vi "SC_schleife_init_JT_2.vi"   [LabVIEW 2016]
uses:
  Global/Global Variables/global.vi
  Global/Global Variables/Data_Display_global.vi
  Instrument_Setup.vi
types:
  T1 = typedef "PSIO.ctl" = cluster{"Address":T2, "Version":enum16{"PS", "IPS"}}
  T2 = typedef "OxfordAddress.ctl" = cluster{"Com Port":i32, "ISOBUS Address":i32, "GPIB Address":i16, "Communication":enum16{"RS232", "ISOBUS", "GPIB", "Gateway"}}
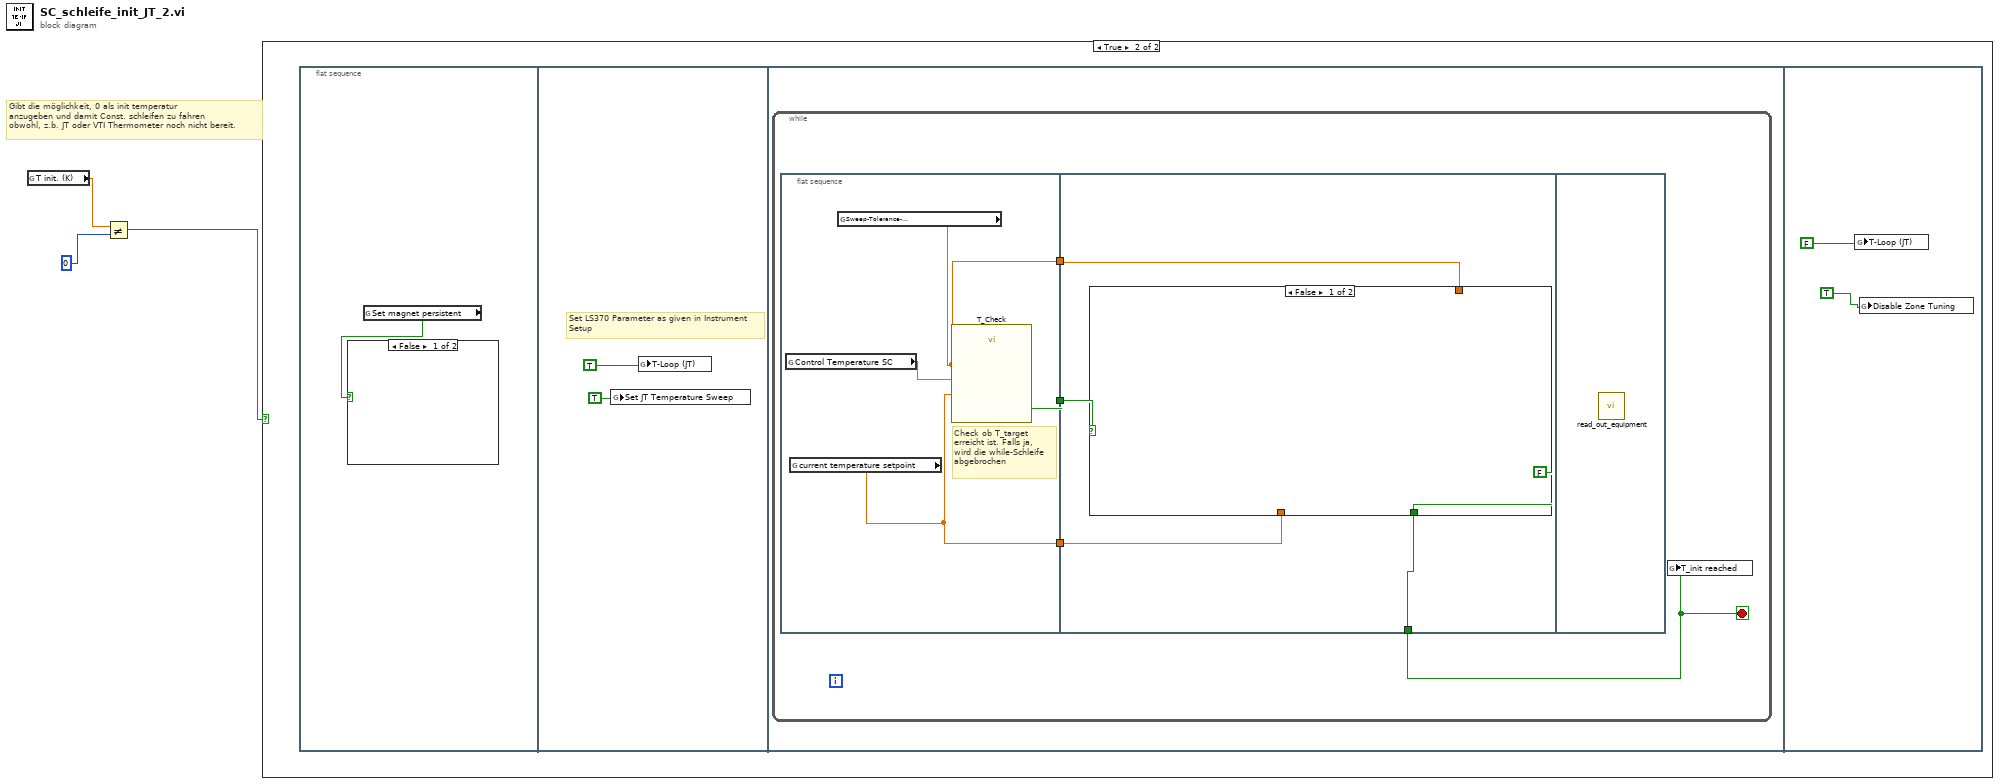
[diagram p0: block diagram]
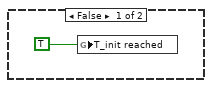
[diagram p2: hidden frame]
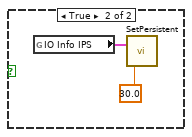
[diagram p3: hidden frame]
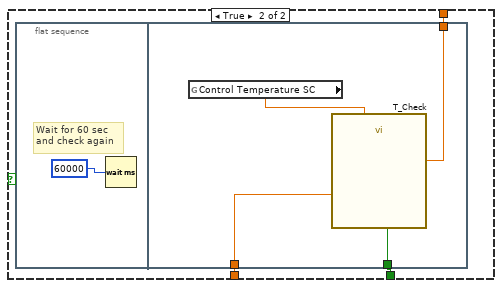
[diagram p4: hidden frame]
diagram:
  # "Gibt die möglichkeit, 0 als init temperatur \nanzugeben und damit Const. schleifen zu fahren\nobwohl, z.b. JT oder VTI Thermometer noch nicht bereit."
  n1 = global read "global.vi" "T init. (K)"() -> (w3:dbl)
  n2 = Not Equal?(x=w3, y=0) -> (x != y?=w1:bool)
  n3 = case shown="True" w1 {
    frame False {
      n4 = global write "Data_Display_global.vi" "T_init reached"(TRUE) -> ()
    }
    frame True {
      n5 = flat-sequence {
        frame #0 {
          n6 = global read "Instrument_Setup.vi" "Set magnet persistent"() -> (w5:bool)
          n7 = case shown="False" w5 {
            frame False {
            }
            frame True {
              n8 = global read "Instrument_Setup.vi" "IO Info IPS"() -> (w6:T1)
              n9 = call "SetPersistent.vi"("Switch Heater Dwell Time"=dbl[unit] 30.0, "IO Info"=w6) -> ()  [unwired: 1 in, 1 out]
            }
          }
        }
        frame #1 {
          # "Set LS370 Parameter as given in Instrument \nSetup"
          n10 = global write "global.vi" "Set JT Temperature Sweep"(TRUE) -> ()
          n11 = global write "global.vi" "T-Loop (JT)"(TRUE) -> ()
        }
        frame #2 {
          n12 = while {
            stop <- w10 stop-if-true
            n13 = flat-sequence {
              tunnel: [w17] -> w13
              tunnel: [w14] -> w12
              tunnel: [w16] -> w11
              tunnel: w13 -> [w21]
              tunnel: w12 -> [w20]
              tunnel: w11 -> [w19]
              tunnel: [w18] -> w10
              frame #0 {
                # "Check ob T_target\nerreicht ist. Falls ja,\nwird die while-Schleife\nabgebrochen"
                n14 = global read "Data_Display_global.vi" "Control Temperature SC"() -> (w15:dbl)
                n15 = global read "Data_Display_global.vi" "current temperature setpoint"() -> (w14:dbl)
                n16 = global read "Instrument_Setup.vi" "Sweep-Tolerance-\nTemperature"() -> (w16:dbl)
                n17 = call "T_Check.vi"("Sweep\nTolerance %"=w16, "T_target (K)"=w14, "T_in"=w15) -> ("= T target"=w17:bool)
              }
              frame #1 {
                n18 = case shown="False" w21 {
                  tunnel: w20 -> [_ w25]
                  tunnel: w19 -> [_ w24]
                  tunnel: [FALSE w23] -> w18
                  frame False {
                  }
                  frame True {
                    n19 = flat-sequence {
                      tunnel: w25 -> [w30]
                      tunnel: w24 -> [w29]
                      tunnel: [w28] -> w23
                      frame #0 {
                        # "Wait for 60 sec\nand check again"
                        n20 = Wait (ms)(milliseconds to wait=60000) -> ()  [unwired: 1 out]
                      }
                      frame #1 {
                        n21 = global read "Data_Display_global.vi" "Control Temperature SC"() -> (w27:dbl)
                        n22 = call "T_Check.vi"("Sweep\nTolerance %"=w29, "T_target (K)"=w30, "T_in"=w27) -> ("= T target"=w28:bool)
                      }
                    }
                  }
                }
              }
              frame #2 {
                n23 = call "read_out_equipment.vi"() -> ()  [unwired: 1 in]
              }
            }
            n24 = global write "Data_Display_global.vi" "T_init reached"(w10) -> ()
          }
        }
        frame #3 {
          n25 = global write "global.vi" "T-Loop (JT)"(FALSE) -> ()
          n26 = global write "global.vi" "Disable Zone Tuning"(TRUE) -> ()
        }
      }
    }
  }
